vi "Set Debug Options.vi"(8 "error in":errorcluster, 9 "infinite FIFO timeouts":bool, 10 "debug":bool, 11 "data sharing framework custom device in":T1 format="%.0x") -> (0 "error out":errorcluster, 3 "data sharing framework custom device out":T1 format="%.0x")   [LabVIEW 2017, in "Data Sharing Framework Custom Device Scripting.lvlib"]
uses:
  Data Sharing Framework Custom Device Scripting.lvlib
  <vilib>/NI Veristand/Custom Device API/Custom Device Item Ref.ctl
  <vilib>/NI Veristand/Custom Device API/Set Item Property (Boolean).vi
  Shared/DSF Shared.lvlib
  <vilib>/NI Veristand/Custom Device API/Custom Device API.lvlib
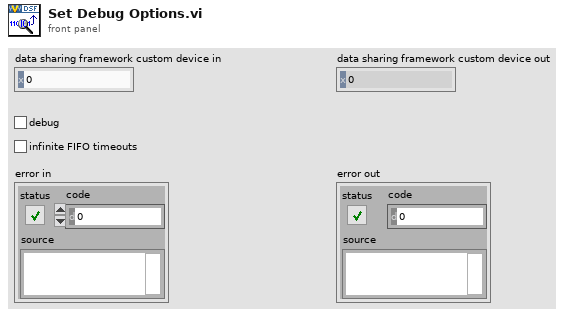
[diagram p1: front panel]
types:
  T1 = typedef "Custom Device API.lvlib/Custom Device Item Ref.ctl" = u64
  T2 = typedef "DSF Core.lvlibp/Framework.lvclass/Framework Options.ctl" = cluster{"FIFO Options":T3, "Thread Options":T4, "Plugin Options":T5, "Performance Options":T6, "Data Server Options":T7}
  T3 = typedef "DSF Core.lvlibp/Framework.lvclass/DSF FIFO Options.ctl" = cluster{"Infinite Timeouts":bool}
  T4 = typedef "DSF Core.lvlibp/Thread.lvclass/Thread Options.ctl" = cluster{"Show FP On Call":bool, "Close FP After Call":bool, "Allow Debugging":bool}
  T5 = typedef "DSF Core.lvlibp/Framework.lvclass/DSF Plugin Options.ctl" = cluster{"Default Components":bool}
  T6 = typedef "DSF Core.lvlibp/DSF Performance Options.ctl" = cluster{"Measure Period":bool, "Measure Rx/Tx Duration":bool}
  T7 = typedef "DSF Core.lvlibp/Framework.lvclass/Data Server Options.ctl" = cluster{"Enable Data Server":bool, "Period":u32}
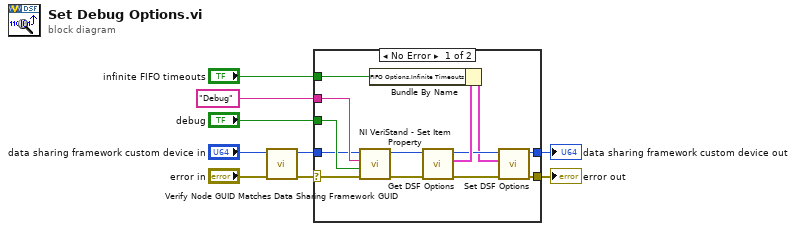
[diagram p0: block diagram]
diagram:
  n1 = call "Verify Node GUID Matches Data Sharing Framework GUID.vi"("error in"="error in", "data sharing framework custom device in"="data sharing framework custom device in") -> ("error out"=w1:errorcluster, "data sharing framework custom device out"=w2:T1)  [unwired: 8 in]
  n2 = case shown="No Error" w1 {
    selector: w1 -> [w10 w23]
    tunnel: "Debug" ("Property Name") -> [w22 _]
    tunnel: "debug" -> [w19 _]
    tunnel: "infinite FIFO timeouts" -> [w17 _]
    tunnel: [w14 w24] -> w6
    tunnel: [w13 w23] -> w5
    tunnel: w2 -> [w11 w24]
    frame No Error {
      n3 = call-poly <vilib>:"NI VeriStand - Set Item Property.vi"("error in (no error)"=w10, "Value"=w19, "Property Name"=w22, "Item Ref in"=w11) -> ("error out"=w20:errorcluster, "Item Ref out"=w21:T1)  [unwired: 5 in, 1 out]
      n4 = call "Get DSF Options.vi"("error in (no error)"=w20, "Item Ref in"=w21) -> ("error out"=w15:errorcluster, "options"=w18:T2, "Item Ref out"=w16:T1)  [unwired: 7 in]
      n5 = Bundle By Name(cluster=w18, "FIFO Options.Infinite Timeouts"=w17) -> (w12:T2)
      n6 = call "Set DSF Options.vi"("error in (no error)"=w15, "options"=w12, "Item Ref in"=w16) -> ("error out"=w13:errorcluster, "Item Ref out"=w14:T1)  [unwired: 7 in]
    }
    frame Error {
    }
  }
  "data sharing framework custom device out" <- w6
  "error out" <- w5
